vi "Run_Core.vi"(0 "Comparison Operations in":refnum<class "Comparison Functions.lvclass">, 11 "error in (no error)":errorcluster) -> (4 "Comparison Operations out":refnum<class "Comparison Functions.lvclass">, 6 "Return":variant, 15 "error out":errorcluster)   [LabVIEW 2019, in "Comparison Functions.lvclass"]
uses:
  Comparison Functions.lvclass
  Comparison Functions.lvclass/Comparison Functions.ctl
  Function List.ctl
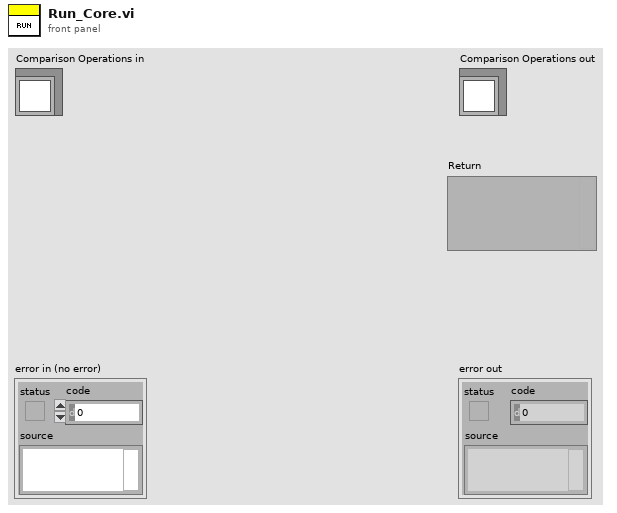
[diagram p1: front panel]
types:
  T1 = typedef "Comparison Functions.lvclass/Function List.ctl" = enum16{"Equal", "Not Equal", "Greater Than", "Less Than", "Greater Than Or Equal", "Lesser Than Or Equal", "Equal To Zero", "Select One", "In Range", "Empty Array", "Empty String", "Not A Number"}
  T2 = typedef "Datatype.ctl" = enum16{"Null", "Numeric", "String", "Bool", "Numeric 1D", "String 1D", "Bool 1D", "Numeric 2D", "String 2D", "Bool 2D", "Variant"}
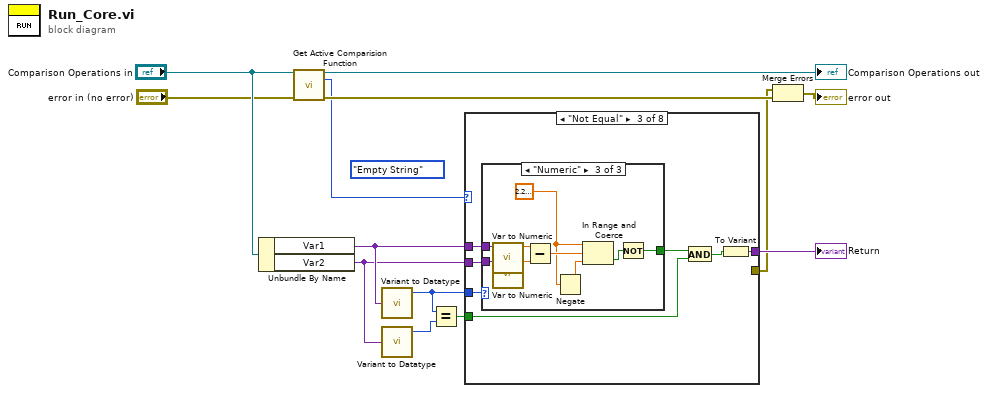
[diagram p0: block diagram]
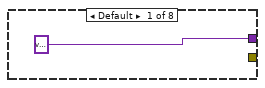
[diagram p2: hidden frame]
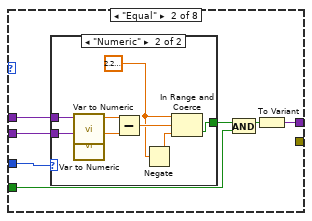
[diagram p3: hidden frame]
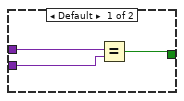
[diagram p4: hidden frame]
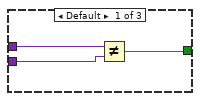
[diagram p5: hidden frame]
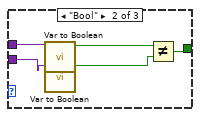
[diagram p6: hidden frame]
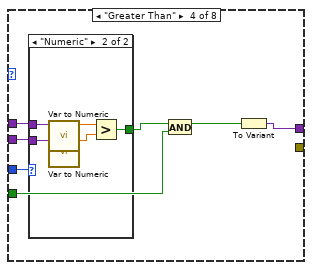
[diagram p7: hidden frame]
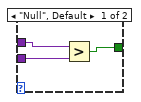
[diagram p8: hidden frame]
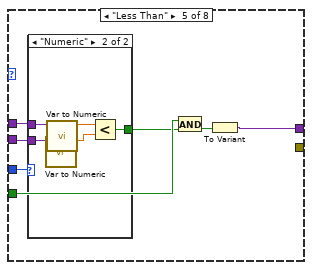
[diagram p9: hidden frame]
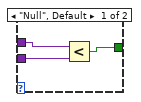
[diagram p10: hidden frame]
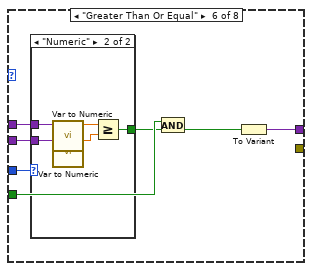
[diagram p11: hidden frame]
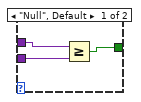
[diagram p12: hidden frame]
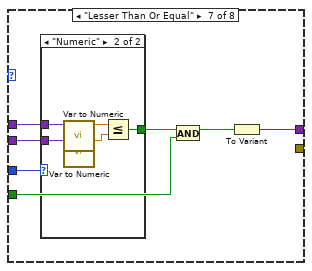
[diagram p13: hidden frame]
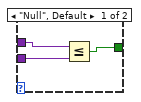
[diagram p14: hidden frame]
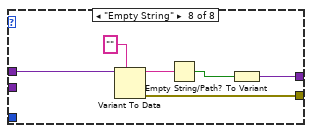
[diagram p15: hidden frame]
diagram:
  (unwired) Function_List."Empty String" ("Function List")
  n1 = Unbundle By Name("Comparison Operations in") -> ("Var1"=w7:variant, "Var2"=w6:variant)
  n2 = call "Get Active Comparision Function.vi"("Comparison Functions in"="Comparison Operations in", "error in (no error)"="error in (no error)") -> ("Comparison Functions out"=→"Comparison Operations out":refnum<class "Comparison Functions.lvclass">, "Function List"=w8:T1, "error out"=w9:errorcluster)  [unwired: 11 in]
  n3 = call "Variant to Datatype.vi"("Variant"=w7) -> ("Datatype"=w3:T2)  [unwired: 2 in, 2 out]
  n4 = call "Variant to Datatype.vi"("Variant"=w6) -> ("Datatype"=w5:T2)  [unwired: 2 in, 2 out]
  n5 = Equal?(x=w3, y=w5) -> (x = y?=w4:bool)
  n6 = case shown="\"Not Equal\"" w8 {
    tunnel: w7 -> [_ w19 w37 w60 w75 w90 w108 w122]
    tunnel: w6 -> [_ w18 w36 w59 w74 w89 w107 _]
    tunnel: [variant ("Variant") w21 w39 w63 w78 w93 w105 w118] -> w13
    tunnel: w4 -> [_ w16 w34 w61 w76 w91 w103 _]
    tunnel: w3 -> [_ w15 w35 w57 w72 w88 w102 _]
    tunnel: [_ _ _ _ _ _ _ w117] -> w1
    frame Default {
    }
    frame "Equal" {
      n7 = case shown="\"Numeric\"" w15 {
        tunnel: [w22 w30] -> w20
        tunnel: w19 -> [w23 w28]
        tunnel: w18 -> [w24 w27]
        frame Default {
          n8 = Equal?(x=w23, y=w24) -> (x = y?=w22:bool)
        }
        frame "Numeric" {
          w29 = 2.220446049250313e-16
          n9 = call "Var to Numeric.vi"("Variant"=w28) -> ("Numeric"=w25:dbl)  [unwired: 10 in]
          n10 = call "Var to Numeric.vi"("Variant"=w27) -> ("Numeric"=w26:dbl)  [unwired: 10 in]
          n11 = Subtract(x=w25, y=w26) -> (x-y=w32:dbl)
          n12 = Negate(x=w29) -> (-x=w31:dbl)
          n13 = In Range and Coerce(upper limit=w29, x=w32, lower limit=w31) -> (In Range?=w30:bool)  [unwired: 1 out]
        }
      }
      n14 = And(x=w20, y=w16) -> (x .and. y?=w17:bool)
      n15 = To Variant(anything=w17) -> (Variant=w21:variant)
    }
    frame "Not Equal" {
      n16 = case shown="\"Numeric\"" w35 {
        tunnel: [w41 w47 w48] -> w33
        tunnel: w36 -> [w42 w45 w52]
        tunnel: w37 -> [w40 w46 w49]
        frame Default {
          n17 = Not Equal?(x=w40, y=w42) -> (x != y?=w41:bool)
        }
        frame "Bool" {
          n18 = call "Var to Boolean.vi"("Variant"=w46) -> ("Boolean"=w44:bool)  [unwired: 10 in]
          n19 = call "Var to Boolean.vi"("Variant"=w45) -> ("Boolean"=w43:bool)  [unwired: 10 in]
          n20 = Not Equal?(x=w44, y=w43) -> (x != y?=w47:bool)
        }
        frame "Numeric" {
          w53 = 2.220446049250313e-16
          n21 = call "Var to Numeric.vi"("Variant"=w49) -> ("Numeric"=w50:dbl)  [unwired: 10 in]
          n22 = call "Var to Numeric.vi"("Variant"=w52) -> ("Numeric"=w51:dbl)  [unwired: 10 in]
          n23 = Subtract(x=w50, y=w51) -> (x-y=w56:dbl)
          n24 = Negate(x=w53) -> (-x=w55:dbl)
          n25 = In Range and Coerce(upper limit=w53, x=w56, lower limit=w55) -> (In Range?=w54:bool)  [unwired: 1 out]
          n26 = Not(x=w54) -> (.not. x?=w48:bool)
        }
      }
      n27 = And(x=w33, y=w34) -> (x .and. y?=w38:bool)
      n28 = To Variant(anything=w38) -> (Variant=w39:variant)
    }
    frame "Greater Than" {
      n29 = case shown="\"Numeric\"" w57 {
        tunnel: w60 -> [w66 w70]
        tunnel: w59 -> [w65 w68]
        tunnel: [w64 w71] -> w58
        frame "Null", Default {
          n30 = Greater?(x=w66, y=w65) -> (0:w64:bool)
        }
        frame "Numeric" {
          n31 = call "Var to Numeric.vi"("Variant"=w70) -> ("Numeric"=w69:dbl)  [unwired: 10 in]
          n32 = call "Var to Numeric.vi"("Variant"=w68) -> ("Numeric"=w67:dbl)  [unwired: 10 in]
          n33 = Greater?(x=w69, y=w67) -> (0:w71:bool)
        }
      }
      n34 = And(x=w58, y=w61) -> (x .and. y?=w62:bool)
      n35 = To Variant(anything=w62) -> (Variant=w63:variant)
    }
    frame "Less Than" {
      n36 = case shown="\"Numeric\"" w72 {
        tunnel: w75 -> [w81 w85]
        tunnel: w74 -> [w80 w84]
        tunnel: [w79 w86] -> w73
        frame "Null", Default {
          n37 = Less?(x=w81, y=w80) -> (x < y?=w79:bool)
        }
        frame "Numeric" {
          n38 = call "Var to Numeric.vi"("Variant"=w84) -> ("Numeric"=w82:dbl)  [unwired: 10 in]
          n39 = call "Var to Numeric.vi"("Variant"=w85) -> ("Numeric"=w83:dbl)  [unwired: 10 in]
          n40 = Less?(x=w83, y=w82) -> (x < y?=w86:bool)
        }
      }
      n41 = And(x=w76, y=w73) -> (x .and. y?=w77:bool)
      n42 = To Variant(anything=w77) -> (Variant=w78:variant)
    }
    frame "Greater Than Or Equal" {
      n43 = case shown="\"Numeric\"" w88 {
        tunnel: w90 -> [w96 w100]
        tunnel: w89 -> [w95 w99]
        tunnel: [w94 w101] -> w87
        frame "Null", Default {
          n44 = Greater Or Equal?(x=w96, y=w95) -> (x >= y?=w94:bool)
        }
        frame "Numeric" {
          n45 = call "Var to Numeric.vi"("Variant"=w100) -> ("Numeric"=w98:dbl)  [unwired: 10 in]
          n46 = call "Var to Numeric.vi"("Variant"=w99) -> ("Numeric"=w97:dbl)  [unwired: 10 in]
          n47 = Greater Or Equal?(x=w98, y=w97) -> (x >= y?=w101:bool)
        }
      }
      n48 = And(x=w91, y=w87) -> (x .and. y?=w92:bool)
      n49 = To Variant(anything=w92) -> (Variant=w93:variant)
    }
    frame "Lesser Than Or Equal" {
      n50 = case shown="\"Numeric\"" w102 {
        tunnel: w108 -> [w111 w115]
        tunnel: w107 -> [w110 w113]
        tunnel: [w109 w116] -> w106
        frame "Null", Default {
          n51 = Less Or Equal?(x=w111, y=w110) -> (x <= y?=w109:bool)
        }
        frame "Numeric" {
          n52 = call "Var to Numeric.vi"("Variant"=w115) -> ("Numeric"=w114:dbl)  [unwired: 10 in]
          n53 = call "Var to Numeric.vi"("Variant"=w113) -> ("Numeric"=w112:dbl)  [unwired: 10 in]
          n54 = Less Or Equal?(x=w114, y=w112) -> (x <= y?=w116:bool)
        }
      }
      n55 = And(x=w106, y=w103) -> (x .and. y?=w104:bool)
      n56 = To Variant(anything=w104) -> (Variant=w105:variant)
    }
    frame "Empty String" {
      n57 = Variant To Data(type="", Variant=w122) -> (data=w120:string, error out=w117:errorcluster)  [unwired: 1 in]
      n58 = Empty String/Path?(string/path=w120) -> (empty?=w119:bool)
      n59 = To Variant(anything=w119) -> (Variant=w118:variant)
    }
  }
  "Return" <- w13
  n60 = Merge Errors(w1, w9) -> (→"error out":errorcluster)
